vi "variantTypeToBoolean.vi"(11 "Type In":i16[](array[numeric])) -> (2 "Boolean":bool=TRUE, 3 "Type Out":i16[](array[numeric]))   [LabVIEW 2011]
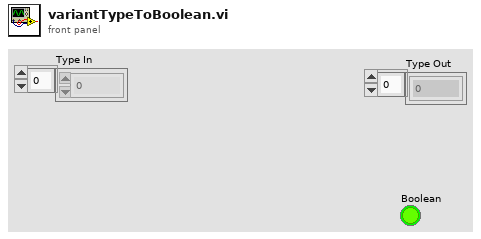
[diagram p1: front panel]
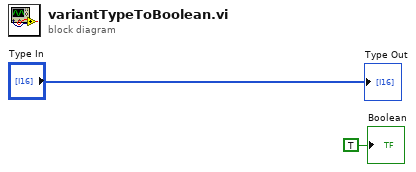
[diagram p0: block diagram]
diagram:
  "Boolean" <- TRUE ("Boolean")
  "Type Out" <- "Type In"
